vi "Construct.vi"(8 "error in":errorcluster, 10 "RT hardware channels":T1[](array[typedef]) {"labels settings for RT"."Label Timestamp Channel Data Reference" format="%.0x"; "labels settings for RT"."Word Initial Raw Value" format="%032.0f"; "labels settings for RT"."Label Disable/Trigger Channel Reference" format="%.0x"; "labels settings for RT"."parameter driver data"."Tx parameter refs" format="%.0x"; "labels settings for RT"."SDI" format="%02b"; "labels settings for RT"."label" format="%.0o"}, 11 "ID":string) -> (0 "error out":errorcluster, 3 "Ballard ARINC-429 Tx Execution Unit out":refnum<class "Tx Scheduled Labels Execution Unit.lvclass">)   [LabVIEW 2020, in "Ballard ARINC 429 Engine.lvlib" / "Implementation.lvlib" / "Tx Scheduled Labels Execution Unit.lvclass"]
uses:
  Tx Scheduled Labels Execution Unit.lvclass
  C:/Git/niveristand-ballard-arinc429-custom-device/Source/Custom Device Support/Engine/Implementation/Execution Unit/Execution Unit.lvclass
  Shared/RT Hardware Channel Settings.ctl
  Shared/RT Label Settings.ctl
  Shared/Label.ctl
  Shared/RT Parameters.ctl
  Shared/Parameter Definition.ctl
  <vilib>/addons/VeriStand Custom Device Scripting APIs/Ballard ARINC 429/Encoding and Decoding/Encoding.ctl
  <vilib>/NI VeriStand/Custom Device API/Custom Device Item Ref.ctl
  Shared/Transfer Type.ctl
  <vilib>/NI VeriStand/Custom Device API/Data Reference.ctl
  Execution Unit/Execution Unit.lvclass/Execution Unit.ctl
  Tx Scheduled Labels Execution Unit.lvclass/Tx Scheduled Labels Execution Unit.ctl
  Execution Unit/Execution Unit.lvclass
  <vilib>/addons/VeriStand Custom Device Scripting APIs/Ballard ARINC 429/Encoding and Decoding/Encoding and Decoding.lvlib
  <vilib>/NI VeriStand/Custom Device API/Custom Device API.lvlib
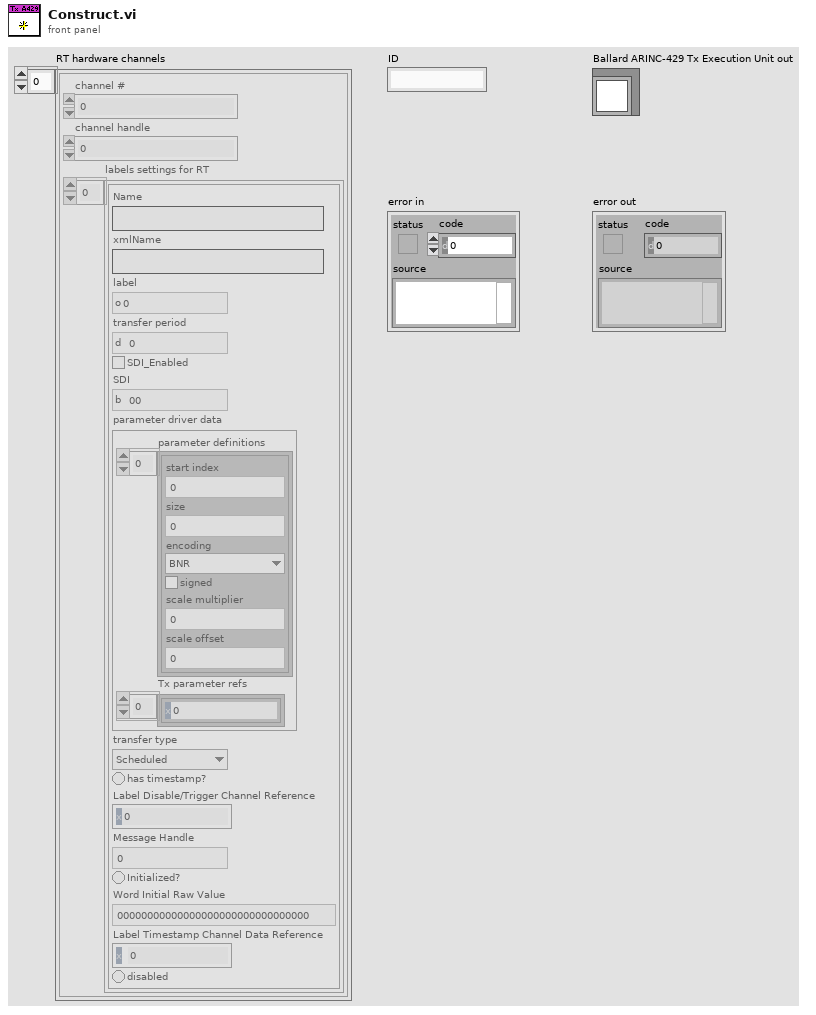
[diagram p1: front panel]
types:
  T1 = typedef "RT Hardware Channel Settings.ctl" = cluster{"channel #":u16, "channel handle":u64, "labels settings for RT":T2[]}
  T2 = typedef "RT Label Settings.ctl" = cluster{"Name":string, "xmlName":string, "label":T3, "transfer period":u32, "SDI_Enabled":bool, "SDI":u8, "parameter driver data":T4, "transfer type":T8, "has timestamp?":bool, "Label Disable/Trigger Channel Reference":T7, "Message Handle":u64, "Initialized?":bool, "Word Initial Raw Value":u32, "Label Timestamp Channel Data Reference":T9, "disabled":bool}
  T3 = typedef "Label.ctl" = u8
  T4 = typedef "RT Parameters.ctl" = cluster{"parameter definitions":T5[], "Tx parameter refs":T7[]}
  T5 = typedef "Parameter Definition.ctl" = cluster{"start index":i32, "size":i32, "encoding":T6, "signed":bool, "scale multiplier":dbl, "scale offset":dbl}
  T6 = typedef "Encoding and Decoding.lvlib/Encoding.ctl" = enum16{"BNR", "BCD", "Discrete"}
  T7 = typedef "Custom Device API.lvlib/Custom Device Item Ref.ctl" = u64
  T8 = typedef "Transfer Type.ctl" = enum16{"Scheduled", "Acyclic", "Block", "Strobe"}
  T9 = typedef "Custom Device API.lvlib/Data Reference.ctl" = i32
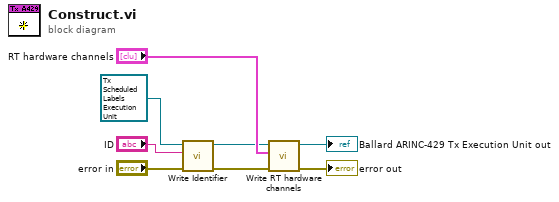
[diagram p0: block diagram]
diagram:
  n1 = call "Write Identifier.vi"("error in (no error)"="error in", "identifier"="ID", "Ballard ARINC-429 Execution Unit in"=refnum<class "Tx Scheduled Labels Execution Unit.lvclass"> refnum ("Ballard ARINC-429 Tx Execution Unit in")) -> ("error out"=w1:errorcluster, "Ballard ARINC-429 Execution Unit out"=w4:refnum<class "Tx Scheduled Labels Execution Unit.lvclass">)  [unwired: 7 in]
  n2 = call "Write RT hardware channels.vi"("error in"=w1, "RT hardware channels"="RT hardware channels", "Ballard ARINC-429 Tx Execution Unit in"=w4) -> ("error out"=→"error out":errorcluster, "Ballard ARINC-429 Tx Execution Unit out"=→"Ballard ARINC-429 Tx Execution Unit out":refnum<class "Tx Scheduled Labels Execution Unit.lvclass">)  [unwired: 7 in]
